vi "To Picture.vi"(8 "error in (no error)":errorcluster, 10 "picture":picture, 11 "Bitmap Canvas in":refnum<class "Bitmap Canvas.lvclass">) -> (0 "error out":errorcluster, 2 "new picture":picture, 3 "Bitmap Canvas out":refnum<class "Bitmap Canvas.lvclass">)   [LabVIEW 2020, in "Glyph Drawer.lvlib" / "Bitmap Canvas.lvclass"]
uses:
  Bitmap Canvas.lvclass
  Bitmap Canvas.lvclass/Bitmap Canvas.ctl
  <vilib>/picture/picture.llb/Draw True-Color Pixmap.vi
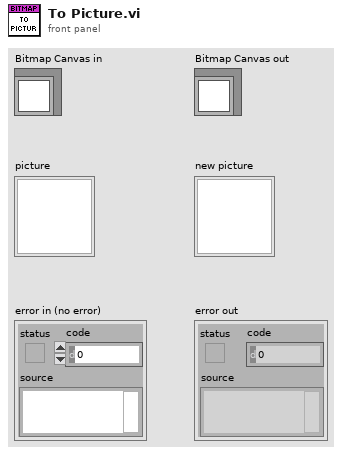
[diagram p1: front panel]
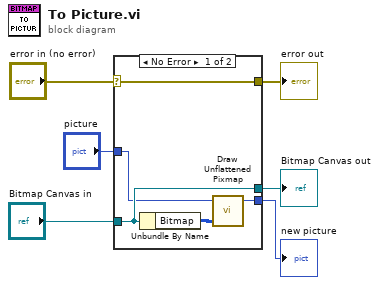
[diagram p0: block diagram]
diagram:
  n1 = case shown="No Error" "error in (no error)" {
    selector: "error in (no error)" -> [w11 w14]
    tunnel: [w11 w14] -> w5
    tunnel: [w10 w13] -> w3
    tunnel: "Bitmap Canvas in" -> [w10 w13]
    tunnel: "picture" -> [w8 w12]
    tunnel: [w7 w12] -> w1
    frame No Error {
      n2 = Unbundle By Name(w10) -> ("Bitmap"=w9:u32[][])
      n3 = call-poly <vilib>:"Draw Unflattened Pixmap.vi"("picture"=w8, "data (RGB format)"=w9) -> ("new picture"=w7:picture)  [unwired: 7 in]
    }
    frame Error {
    }
  }
  "error out" <- w5
  "Bitmap Canvas out" <- w3
  "new picture" <- w1
